vi "Write Sample name.vi"(8 "error in (no error)":errorcluster, 10 "Sample name":string, 11 "Data3D in":refnum<class "Data3D.lvclass">) -> (0 "error out":errorcluster, 3 "Data3D out":refnum<class "Data3D.lvclass">)   [LabVIEW 2014, in "Data3D.lvclass"]
uses:
  Data3D.lvclass
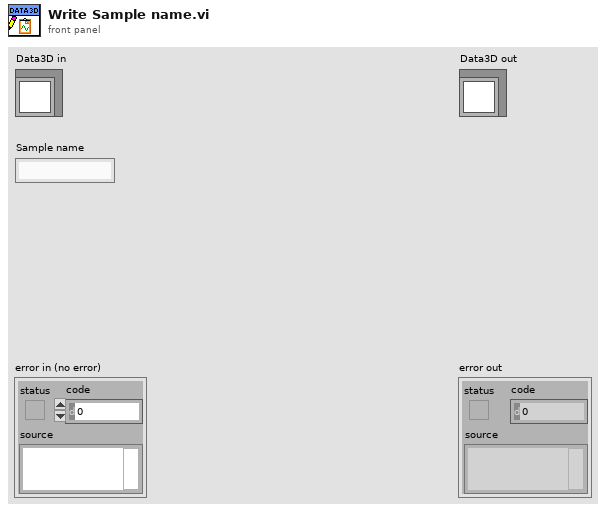
[diagram p1: front panel]
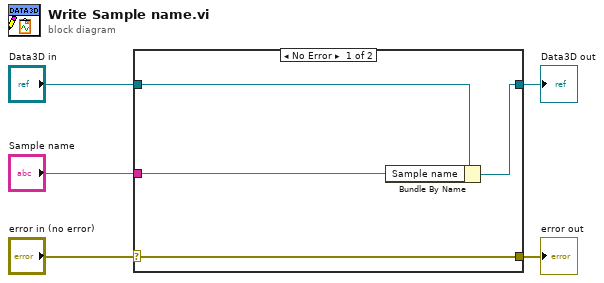
[diagram p0: block diagram]
diagram:
  n1 = case shown="No Error" "error in (no error)" {
    selector: "error in (no error)" -> [w9 w10]
    tunnel: [w9 w10] -> w4
    tunnel: [w7 w11] -> w2
    tunnel: "Data3D in" -> [w8 w11]
    tunnel: "Sample name" -> [w6 _]
    frame No Error {
      n2 = Bundle By Name(cluster=w8, "Sample name"=w6) -> (w7:refnum<class "Data3D.lvclass">)
    }
    frame Error {
    }
  }
  "error out" <- w4
  "Data3D out" <- w2
